vi "PS_Global.vi"() -> ()   [LabVIEW 2011]
panel:
  in  "Laser Calibration Filename":path=path "C:/Users/He3RHIC/Desktop/PolStat/laser data/laser_set.lvm"
  in  "LCR Calibration Filename":path=path "C:/Users/He3RHIC/Desktop/PolStat/lcr data/lcr_cal.lvm"
  in  "Polarization Filename":path=path "C:/Users/He3RHIC/Desktop/PolStat/Data/PS_data.lvm"
  in  "LCR Trigger Port 2":tag="Dev1/port1/line4"
  in  "Liquid Crystal Controller Port 2":refnum<visa-resource-name>="COM7"
  in  "BK Signal Generator Port":refnum<visa-resource-name>="COM7"
  out "Path":path
  out "Laser Peak Progress":u8(slide) scale=0.0..100.0
  in  "Liquid Crystal Controller Port":refnum<visa-resource-name>="COM3"
  out "Calibration Progress":u8(slide) scale=0.0..100.0
  in  "Shutter Control Port":tag="Dev1/port1/line1"
  in  "Discharge Control Port":tag="Dev1/port1/line2"
  in  "LCR Trigger Port 1":tag="Dev1/port1/line0"
  in  "Plasma Ball Control":tag="Dev1/port1/line3"
  in  "Log File":path=path "C:/Users/He3RHIC/Desktop/PolStat/PS_LOG.txt"
  out "Signal Offset: Laser Off":dbl
  out "Signal Offset: Laser On":dbl
  in  "Laser State":bool
  in  "Laser Modulation Channel":tag="Dev1/ao0"
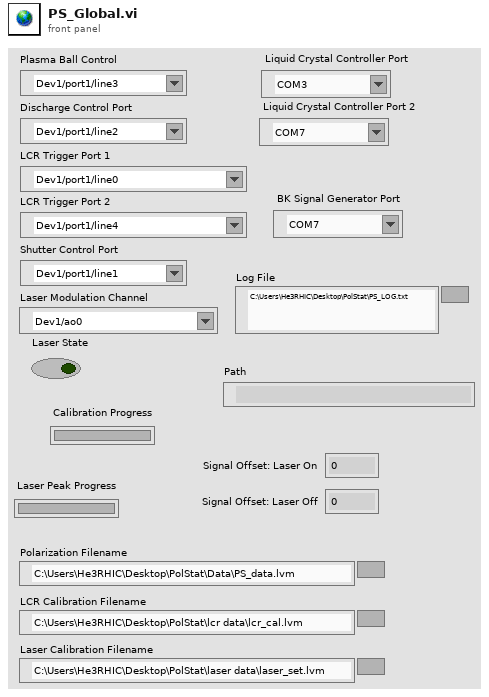
[diagram p1: front panel]
diagram:
